vi "Handle MissionOp Waypoint.vi"(8 "error in (no error)":errorcluster, 11 "RDS Mission Controller Actor in":refnum<class "RDS Mission Controller Actor.lvclass">) -> (0 "error out":errorcluster, 3 "RDS Mission Controller Actor out":refnum<class "RDS Mission Controller Actor.lvclass">)   [LabVIEW 2015, in "RDS Mission Controller Actor.lvlib" / "RDS Mission Controller Actor.lvclass"]
uses:
  RDS Mission Controller Actor.lvclass
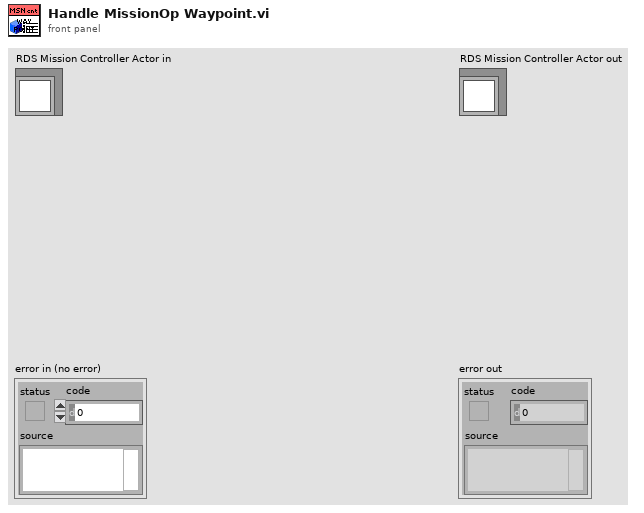
[diagram p1: front panel]
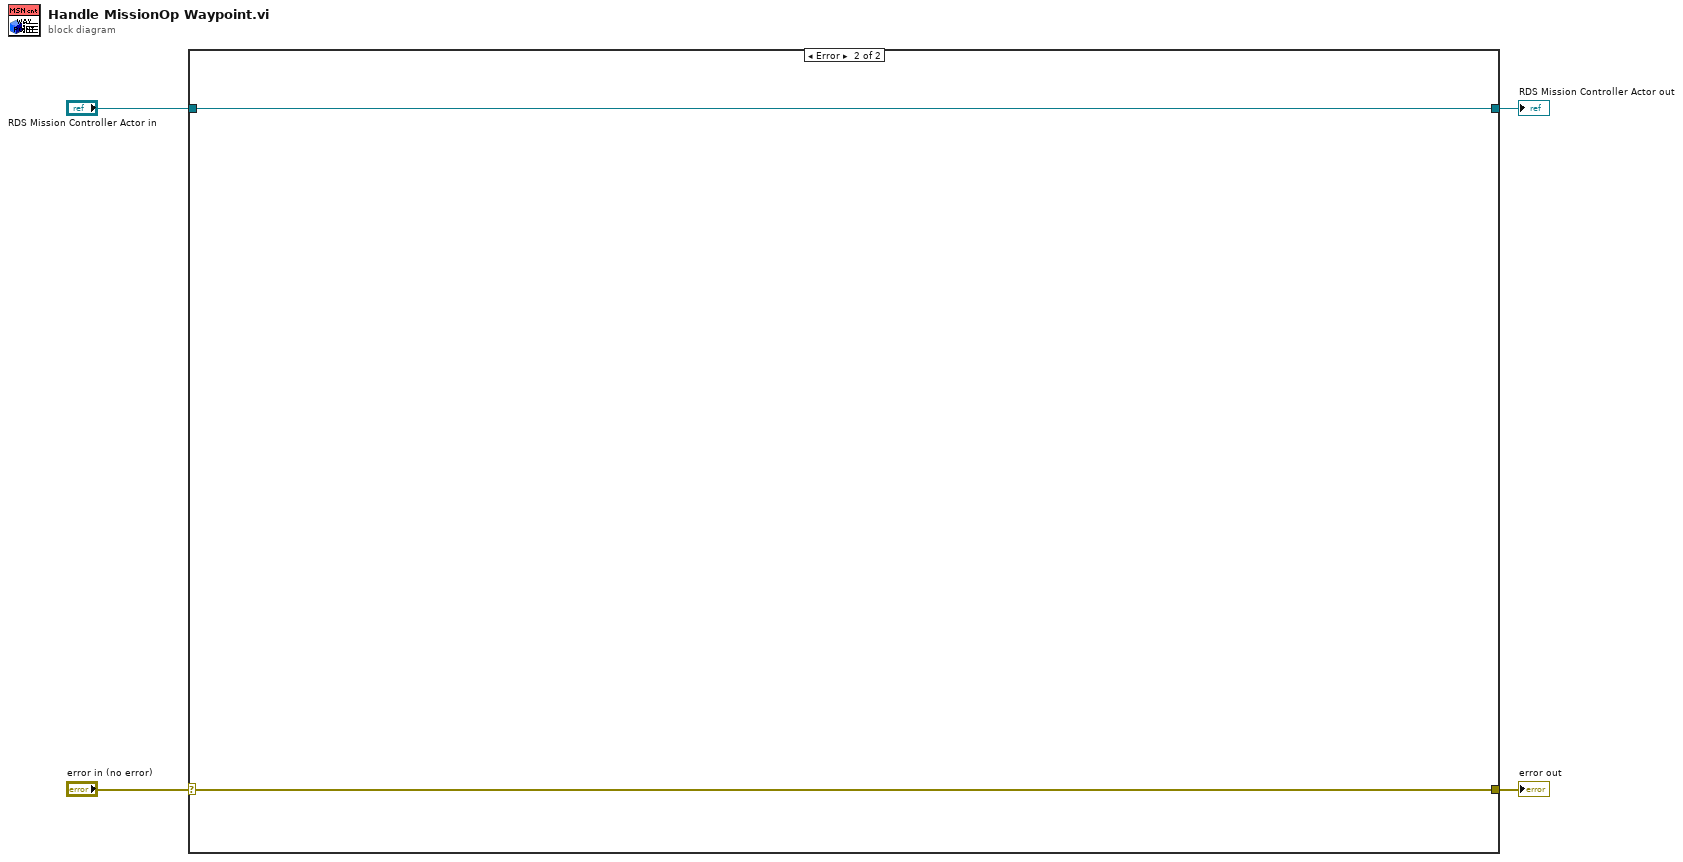
[diagram p0: block diagram]
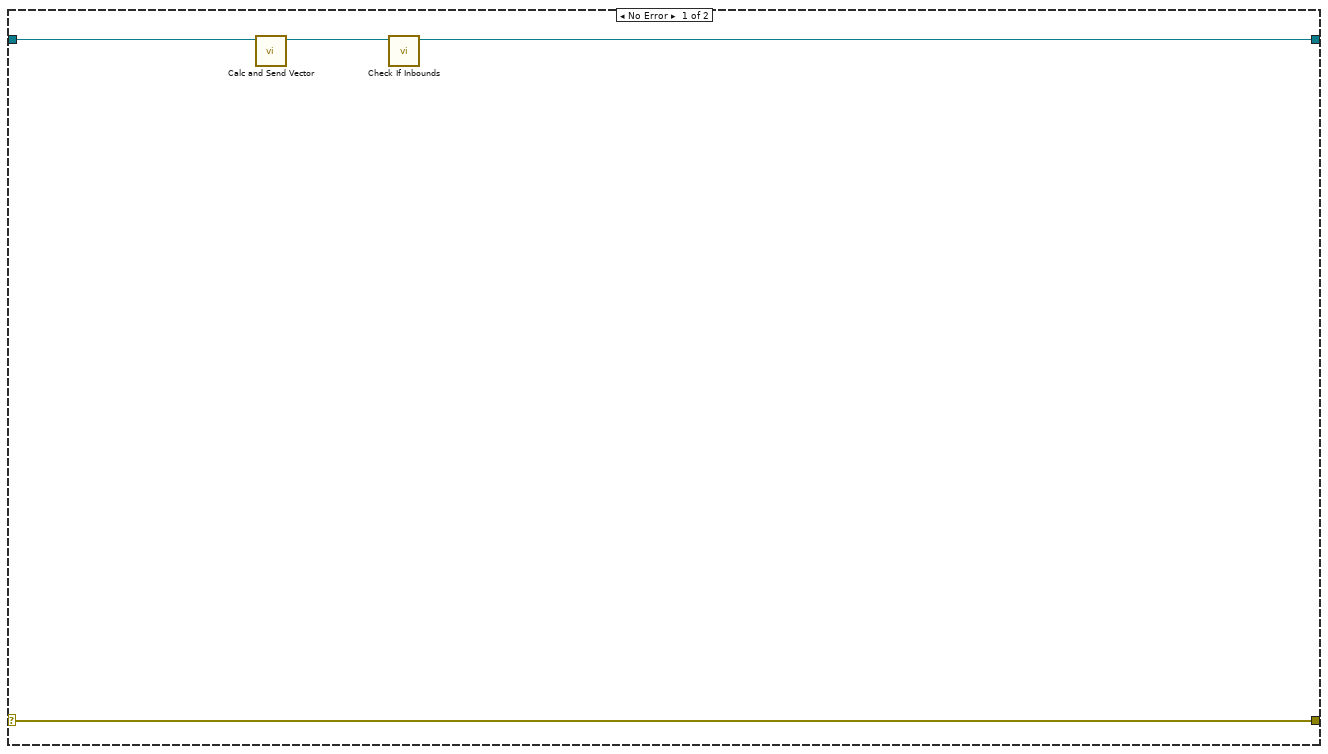
[diagram p2: hidden frame]
diagram:
  n1 = case shown="Error" "error in (no error)" {
    selector: "error in (no error)" -> [w8 w10]
    tunnel: [w8 w10] -> w3
    tunnel: [w5 w9] -> w1
    tunnel: "RDS Mission Controller Actor in" -> [w7 w9]
    frame No Error {
      n2 = call "Calc and Send Vector.vi"("RDS Mission Controller Actor in"=w7) -> ("RDS Mission Controller Actor out"=w6:refnum<class "RDS Mission Controller Actor.lvclass">)  [unwired: 9 in, 1 out]
      n3 = call "Check If Inbounds.vi"("RDS Mission Controller Actor in"=w6) -> ("RDS Mission Controller Actor out"=w5:refnum<class "RDS Mission Controller Actor.lvclass">)  [unwired: 9 in, 1 out]
    }
    frame Error {
    }
  }
  "error out" <- w3
  "RDS Mission Controller Actor out" <- w1
